vi "Actor Core.vi"(8 "error in":errorcluster, 11 "[MDI] Child in":refnum<class "[MDI] Child.lvclass">) -> (0 "error out":errorcluster, 3 "Actor out":refnum<class "Actor.lvclass">)   [LabVIEW 2020, in "[MDI] Child.lvlib" / "[MDI] Child.lvclass"]
doc: "(<B>Filename</B>: Actor Framework.lvlib:Actor.lvclass:Actor Core.vi)\n\nReceives messages to the actor, reacts to them, and initiates any error handling that may shut the actor down.\n\nDescendant classes may override this VI to append parallel tasks for the actor to complete while it handles messages. Overrides use the Call Parent Class Method node."
uses:
  [MDI] Child.lvclass
  <vilib>/ActorFramework/Actor/Actor.lvclass
  [MDI] Child.lvclass/[MDI] Child.ctl
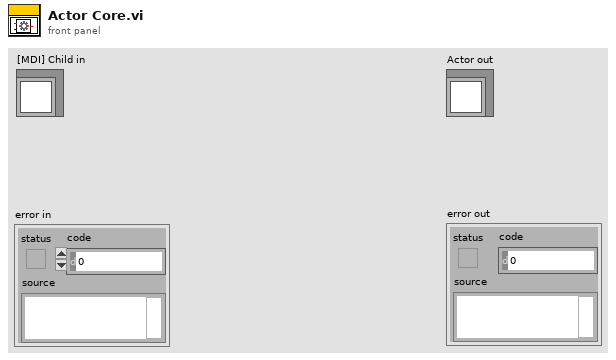
[diagram p1: front panel]
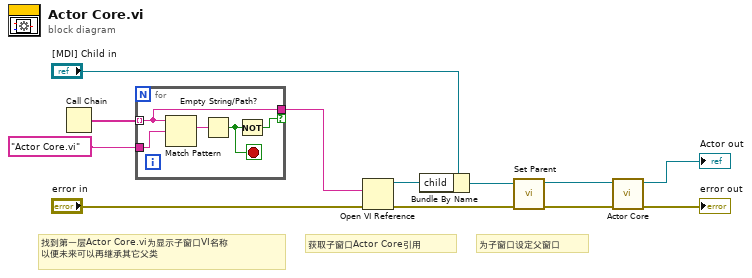
[diagram p0: block diagram]
diagram:
  # "为子窗口设定父窗口"
  # "获取子窗口Actor Core引用"
  # "找到第一层Actor Core.vi为显示子窗口VI名称\n以便未来可以再继承其它父类"
  n1 = Call Chain() -> (call chain=w4:string[])
  n2 = for {
    tunnel: w4 -> [w14] mode=indexing
    tunnel: "Actor Core.vi" ("regular expression") -> [w17]
    tunnel: [w14] -> w1 if=w15
    stop <- w13 stop-if-true
    n3 = Match Pattern(string=w14, regular expression=w17) -> (match substring=w16:string)  [unwired: 1 in, 3 out]
    n4 = Empty String/Path?(string/path=w16) -> (empty?=w13:bool)
    n5 = Not(x=w13) -> (.not. x?=w15:bool)
  }
  n6 = Open VI Reference(vi path=w1, error in (no error)="error in") -> (vi reference=w9:refnum<vi>, error out=w8:errorcluster)  [unwired: 4 in]
  n7 = Bundle By Name(cluster="[MDI] Child in", "child"=w9) -> (w6:refnum<class "[MDI] Child.lvclass">)
  n8 = call "Set Parent.vi"("error in (no error)"=w8, "[MDI] Child in"=w6) -> ("error out"=w7:errorcluster, "[MDI] Child out"=w5:refnum<class "[MDI] Child.lvclass">)  [unwired: 8 in]
  n9 = call-parent "Actor Core.vi"("error in"=w7, "Actor in"=w5) -> ("error out"=→"error out":errorcluster, "Actor out"=→"Actor out":refnum<class "Actor.lvclass">)  [unwired: 8 in]
